vi "Read Frame.vi"(8 "error in (no error)":errorcluster, 9 "Timeout ms":i32, 11 "WebSocket Client in":refnum<class "WebSocket Client.lvclass">) -> (0 "error out":errorcluster, 1 "Remaining  Timeout":i32, 2 "Message Frame":T1, 3 "WebSocket Client out":refnum<class "WebSocket Client.lvclass">)   [LabVIEW 2020, in "HTTP Server.lvlib" / "WebSocket Client.lvclass"]
uses:
  WebSocket Client.lvclass
  WebSocket Client.lvclass/WebSocket Client.ctl
  OpCode.ctl
  Message Frame.ctl
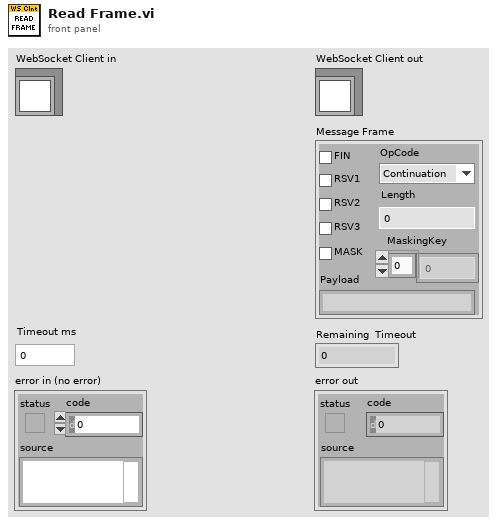
[diagram p1: front panel]
types:
  T1 = typedef "HTTP Server.lvlib/WebSocket Client.lvclass/Message Frame.ctl" = cluster{"FIN":bool, "RSV1":bool, "RSV2":bool, "RSV3":bool, "MASK":bool, "OpCode":T2, "Length":u64, "MaskingKey":u8[], "Payload":string}
  T2 = typedef "HTTP Server.lvlib/WebSocket Client.lvclass/OpCode.ctl" = enum8{"Continuation", "Text", "Binary", "Reserved3", "Reserved4", "Reserved5", "Reserved6", "Reserved7", "Close", "Ping", "Pong", "ReservedB", "ReservedC", "ReservedD", "ReservedE", "ReservedF"}
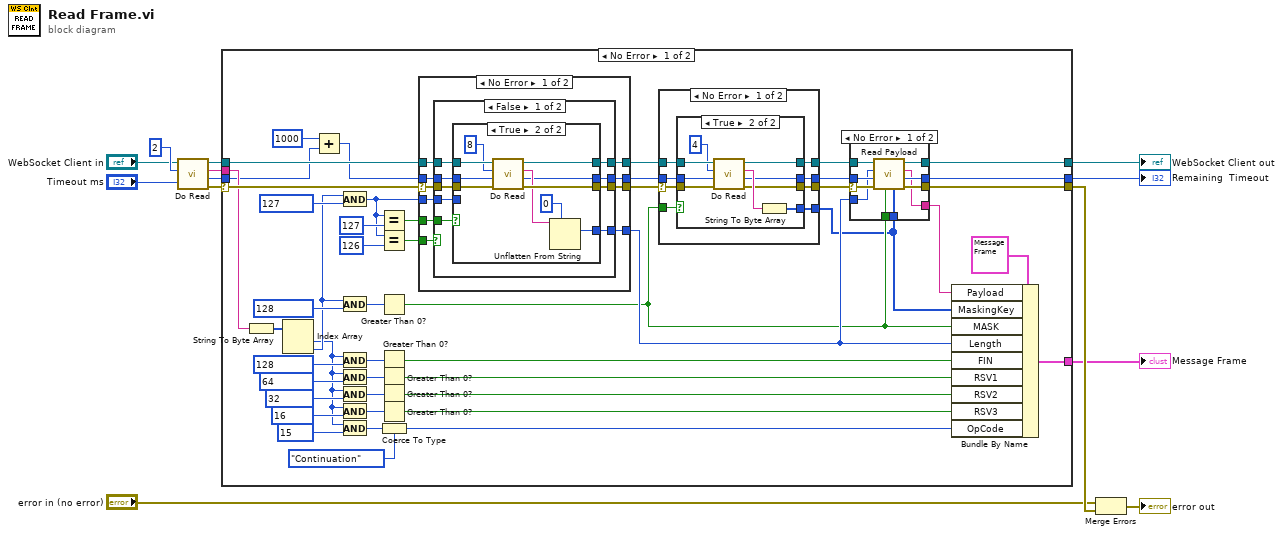
[diagram p0: block diagram]
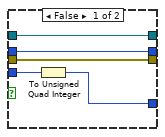
[diagram p5: hidden frame]
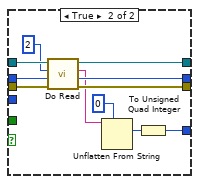
[diagram p6: hidden frame]
diagram:
  n1 = call "Do Read.vi"("Timeout ms"="Timeout ms", "Count"=2, "WebSocket Client in"="WebSocket Client in") -> ("error out"=w11:errorcluster, "Remaining  Timeout"=w10:i32, "Data"=w12:string, "WebSocket Client out"=w9:refnum<class "WebSocket Client.lvclass">)  [unwired: 5 in]
  n2 = case shown="No Error" w11 {
    selector: w11 -> [w61 w146]
    tunnel: w12 -> [w60 _]
    tunnel: w10 -> [w16 w147]
    tunnel: w9 -> [w31 w148]
    tunnel: [w23 w148] -> w4
    tunnel: [w22 w146] -> w7
    tunnel: [w21 w147] -> w8
    tunnel: [w27 _] -> w3
    frame No Error {
      n3 = String To Byte Array(string=w60) -> (unsigned byte array=w59:u8[])
      n4 = Index Array(array=w59) -> (element #1=w50:u8, element #2=w55:u8)  [unwired: 2 in]
      n5 = Add(x=1000, y=w16) -> (x+y=w15:i32)
      n6 = And(x=w55, y=u8 127) -> (x .and. y?=w32:u8)
      n7 = And(x=w55, y=u8 128) -> (x .and. y?=w45:u8)
      n8 = And(x=w50, y=u8 128) -> (x .and. y?=w46:u8)
      n9 = And(x=w50, y=u8 64) -> (x .and. y?=w47:u8)
      n10 = And(x=w50, y=u8 32) -> (x .and. y?=w48:u8)
      n11 = And(x=w50, y=u8 16) -> (x .and. y?=w49:u8)
      n12 = And(x=w50, y=u8 15) -> (x .and. y?=w39:u8)
      n13 = Equal?(x=w32, y=u8 127) -> (x = y?=w34:bool)
      n14 = Equal?(x=w32, y=u8 126) -> (x = y?=w33:bool)
      n15 = Greater Than 0?(x=w45) -> (x > 0?=w18:bool)
      n16 = Greater Than 0?(x=w46) -> (x > 0?=w43:bool)
      n17 = Greater Than 0?(x=w47) -> (x > 0?=w42:bool)
      n18 = Greater Than 0?(x=w48) -> (x > 0?=w41:bool)
      n19 = Greater Than 0?(x=w49) -> (x > 0?=w40:bool)
      n20 = Coerce To Type(0:w39, 1:OpCode."Continuation" ("OpCode")) -> (2:w38:T2)
      n21 = case shown="No Error" w61 {
        selector: w61 -> [w106 w143]
        tunnel: w15 -> [w107 w144]
        tunnel: w34 -> [w105 _]
        tunnel: w33 -> [w104 _]
        tunnel: w32 -> [w103 _]
        tunnel: w31 -> [w102 w145]
        tunnel: [w101 w143] -> w30
        tunnel: [w100 w144] -> w29
        tunnel: [w99 w145] -> w28
        tunnel: [w98 _] -> w19
        frame No Error {
          n22 = case shown="False" w104 {
            tunnel: w103 -> [w116 _]
            tunnel: w102 -> [w115 w142]
            tunnel: w107 -> [w114 w141]
            tunnel: w106 -> [w113 w140]
            tunnel: w105 -> [w112 _]
            tunnel: [w111 w133] -> w98
            tunnel: [w110 w136] -> w101
            tunnel: [w109 w137] -> w100
            tunnel: [w108 w138] -> w99
            frame False {
              n23 = case shown="True" w112 {
                tunnel: w116 -> [w121 _]
                tunnel: w115 -> [w119 w131]
                tunnel: w114 -> [w118 w130]
                tunnel: w113 -> [w117 w129]
                tunnel: [w120 w126] -> w111
                tunnel: [w117 w125] -> w110
                tunnel: [w118 w123] -> w109
                tunnel: [w119 w122] -> w108
                frame False {
                  n24 = To Unsigned Quad Integer(1:w121) -> (0:w120:u64)
                }
                frame True {
                  n25 = call "Do Read.vi"("error in (no error)"=w129, "Timeout ms"=w130, "Count"=8, "WebSocket Client in"=w131) -> ("error out"=w125:errorcluster, "Remaining  Timeout"=w123:i32, "Data"=w124:string, "WebSocket Client out"=w122:refnum<class "WebSocket Client.lvclass">)  [unwired: 4 in]
                  n26 = Unflatten From String(type=u64 0 ("Count"), binary string=w124) -> (value=w126:u64)  [unwired: 3 in, 2 out]
                }
              }
            }
            frame True {
              n27 = call "Do Read.vi"("error in (no error)"=w140, "Timeout ms"=w141, "Count"=2, "WebSocket Client in"=w142) -> ("error out"=w136:errorcluster, "Remaining  Timeout"=w137:i32, "Data"=w132:string, "WebSocket Client out"=w138:refnum<class "WebSocket Client.lvclass">)  [unwired: 4 in]
              n28 = Unflatten From String(type=u16 0 ("Count"), binary string=w132) -> (value=w134:u16)  [unwired: 3 in, 2 out]
              n29 = To Unsigned Quad Integer(1:w134) -> (0:w133:u64)
            }
          }
        }
        frame Error {
        }
      }
      n30 = case shown="No Error" w30 {
        selector: w30 -> [w82 w97]
        tunnel: w29 -> [w81 w96]
        tunnel: w28 -> [w80 w95]
        tunnel: w18 -> [w79 _]
        tunnel: [w78 _] -> w17
        tunnel: [w77 w95] -> w26
        tunnel: [w76 w97] -> w25
        tunnel: [w75 w96] -> w24
        frame No Error {
          n31 = case shown="True" w79 {
            tunnel: w82 -> [w83 w92]
            tunnel: w81 -> [w84 w93]
            tunnel: w80 -> [w85 w94]
            tunnel: [_ w89] -> w78
            tunnel: [w83 w88] -> w76
            tunnel: [w85 w87] -> w77
            tunnel: [w84 w86] -> w75
            frame False {
            }
            frame True {
              n32 = call "Do Read.vi"("error in (no error)"=w92, "Timeout ms"=w93, "Count"=4, "WebSocket Client in"=w94) -> ("error out"=w88:errorcluster, "Remaining  Timeout"=w86:i32, "Data"=w90:string, "WebSocket Client out"=w87:refnum<class "WebSocket Client.lvclass">)  [unwired: 4 in]
              n33 = String To Byte Array(string=w90) -> (unsigned byte array=w89:u8[])
            }
          }
        }
        frame Error {
        }
      }
      n34 = case shown="No Error" w25 {
        selector: w25 -> [w69 w73]
        tunnel: w26 -> [w71 w72]
        tunnel: w24 -> [w70 w74]
        tunnel: [w64 w72] -> w23
        tunnel: [w65 w73] -> w22
        tunnel: [w63 w74] -> w21
        tunnel: [w62 _] -> w20
        tunnel: w19 -> [w68 _]
        tunnel: w18 -> [w67 _]
        tunnel: w17 -> [w66 _]
        frame No Error {
          n35 = call "Read Payload.vi"("MaskingKey"=w66, "Mask"=w67, "error in (no error)"=w69, "Timeout ms"=w70, "Count"=w68, "WebSocket Client in"=w71) -> ("error out"=w65:errorcluster, "Remaining  Timeout"=w63:i32, "Payload"=w62:string, "WebSocket Client out"=w64:refnum<class "WebSocket Client.lvclass">)  [unwired: 2 in]
        }
        frame Error {
        }
      }
      n36 = Bundle By Name(cluster=T1 {"FIN"=FALSE, "RSV1"=FALSE, "RSV2"=FALSE, "RSV3"=FALSE, "MASK"=FALSE, "OpCode"=enum."Continuation", "Length"=0, "MaskingKey"=[], "Payload"=""} ("Message Frame"), "Payload"=w20, "MaskingKey"=w17, "MASK"=w18, "Length"=w19, "FIN"=w43, "RSV1"=w42, "RSV2"=w41, "RSV3"=w40, "OpCode"=w38) -> (w27:T1)
    }
    frame Error {
    }
  }
  "WebSocket Client out" <- w4
  "Remaining  Timeout" <- w8
  "Message Frame" <- w3
  n37 = Merge Errors("error in (no error)", w7) -> (→"error out":errorcluster)
